vi "trapezoidal.vi"(0 "%Subida":dbl, 1 "%Alto":dbl, 2 "%Descida":dbl, 3 "%Baixo":dbl, 4 "Amplitude":dbl) -> (7 "Waveform Graph":dbl[](graph))   [LabVIEW 2017]
uses:
  <vilib>/Analysis/1siggen.llb/Ramp Pattern by Samples.vi
  <vilib>/Analysis/NI_AALBase.lvlib
panel:
  out "appended array":dbl[](array[numeric])
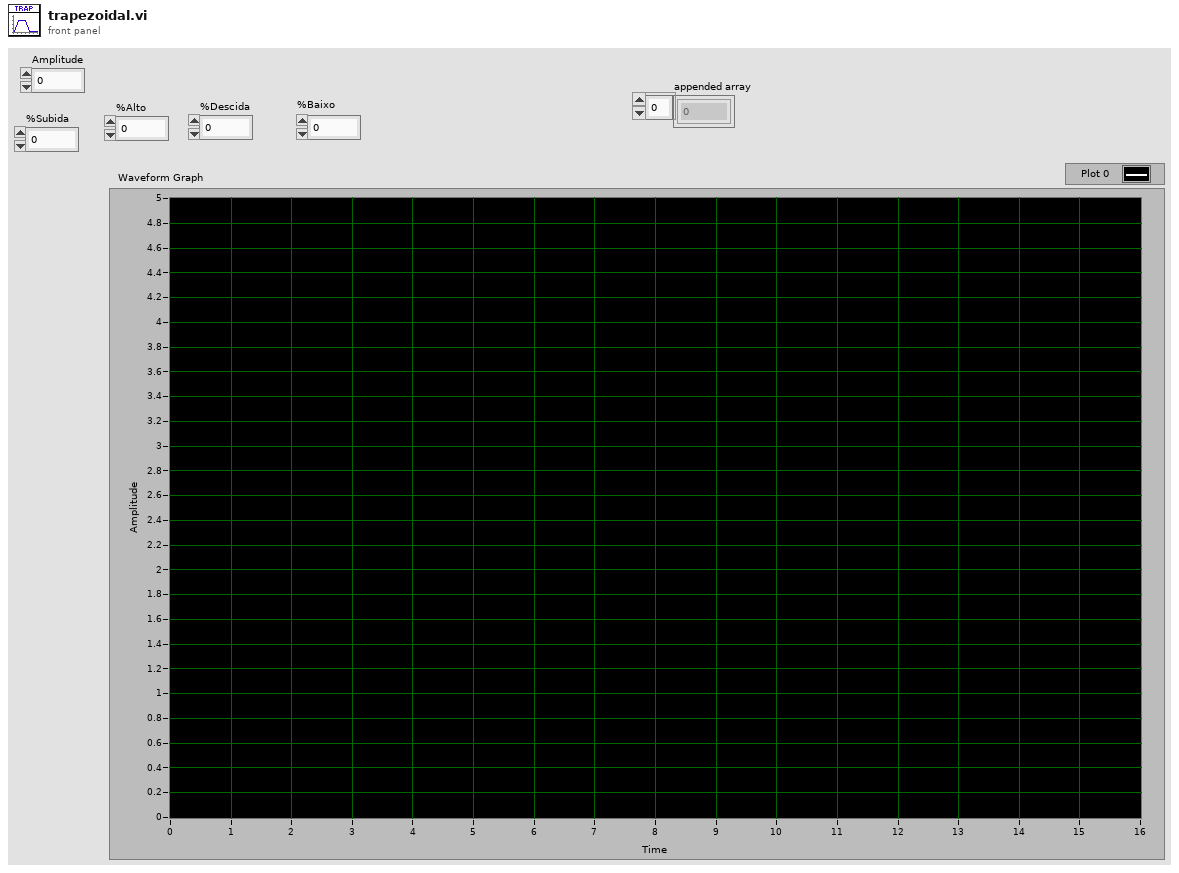
[diagram p1: front panel]
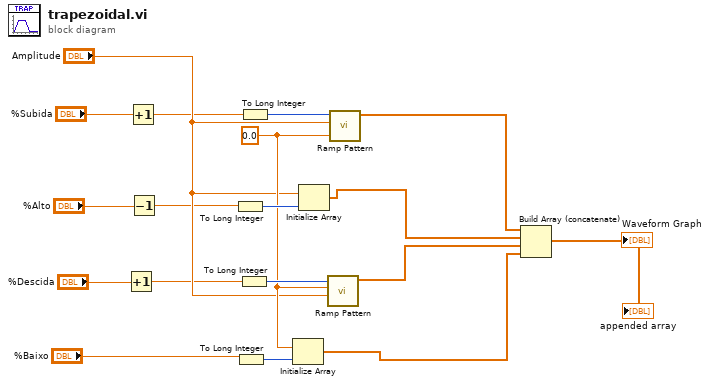
[diagram p0: block diagram]
diagram:
  w9 = 0.0 ("start")
  n1 = Increment(x="%Descida") -> (x+1=w2:dbl)
  n2 = Increment(x="%Subida") -> (x+1=w6:dbl)
  n3 = Decrement(x="%Alto") -> (x-1=w4:dbl)
  n4 = To Long Integer(number=w4) -> (32bit integer=w14:i32)
  n5 = To Long Integer(number="%Baixo") -> (32bit integer=w12:i32)
  n6 = To Long Integer(number=w2) -> (32bit integer=w17:i32)
  n7 = To Long Integer(number=w6) -> (32bit integer=w18:i32)
  n8 = Initialize Array(w9, w12) -> (w11:dbl[])
  n9 = Initialize Array("Amplitude", w14) -> (w13:dbl[])
  n10 = call-poly <vilib>:"Ramp Pattern.vi"("start"="Amplitude", "end"=w9, "samples"=w17) -> ("Ramp Pattern"=w15:dbl[])  [unwired: 7 in, 1 out]
  n11 = call-poly <vilib>:"Ramp Pattern.vi"("start"=w9, "end"="Amplitude", "samples"=w18) -> ("Ramp Pattern"=w16:dbl[])  [unwired: 7 in, 1 out]
  n12 = Build Array (concatenate)(w16, w13, w15, w11) -> (→"Waveform Graph" →"appended array":dbl[])
